vi "Entry.vi"(8 "error in (no error)":errorcluster, 11 "New State":refnum<class "State3.lvclass">) -> (0 "error out":errorcluster, 3 "State out":refnum<class "State3.lvclass">)   [LabVIEW 2025, in "Demo_States.lvlib" / "State3.lvclass"]
doc: "This is an abstract method. Override this method to define the behavior when you enter the state."
uses:
  State3.lvclass
  Demo_States/Demo_States.lvclass
  State3.lvclass/State3.ctl
  C:/Users/halstead_rideriver/Documents/Labview_Practice/ATM_Machine_Actor Framework/ATM_ACTORFW/Demo_States/Demo_States/Demo_States.lvclass
  C:/Program Files (x86)/National Instruments/LabVIEW 2025/vi.lib/ni/Actors/State Actor/State Actor/State Actor.lvclass
  C:/Program Files (x86)/National Instruments/LabVIEW 2025/vi.lib/ActorFramework/Actor/Actor.lvclass
  C:/Users/halstead_rideriver/Documents/Labview_Practice/ATM_Machine_Actor Framework/ATM_ACTORFW/Demo_States/State3/State3.lvclass
  demo Messages/Log State Msg/Log State Msg.lvclass
  <vilib>/ActorFramework/Actor/Actor.lvclass
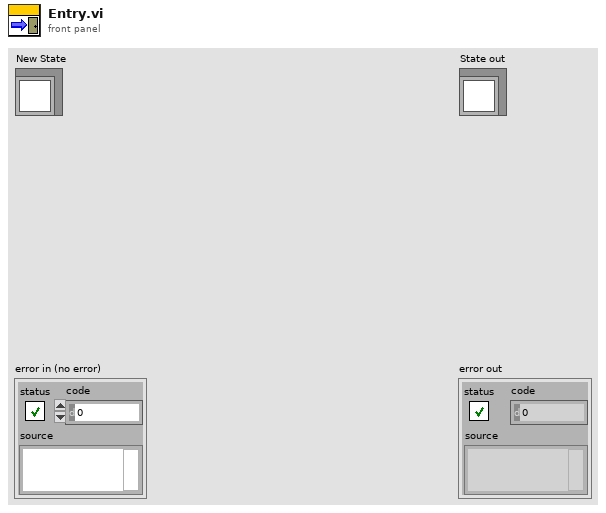
[diagram p1: front panel]
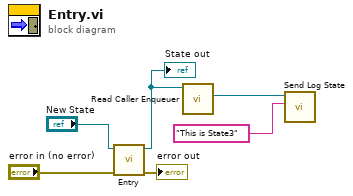
[diagram p0: block diagram]
diagram:
  n1 = call-parent "Entry.vi"("error in (no error)"="error in (no error)", "New State"="New State") -> ("error out"=→"error out":errorcluster, "State out"=w1:refnum<class "State3.lvclass">)  [unwired: 8 in]
  "State out" <- w1
  n2 = call <vilib>:"Read Caller Enqueuer.vi"("Actor"=w1) -> ("Caller Enqueuer"=w3:refnum<class "Message Enqueuer.lvclass">)  [unwired: 10 in]
  n3 = call "Send Log State.vi"("State"="This is State3", "Message Enqueuer"=w3) -> ()  [unwired: 8 in, 2 out]
